vi "ziModGetNextNode.vi"(8 "Error In":errorcluster, 11 "ModHandle In":T4 {"ModHandle" format="0x%08x"; "Conn" format="0x%08x"}) -> (0 "Error Out":errorcluster, 2 "ModResults":T1, 3 "ModHandle Out":T4 {"ModHandle" format="0x%08x"; "Conn" format="0x%08x"}, 4 "NoData":bool)   [LabVIEW 2018, in "Zurich Instruments LabOne.lvlib"]
doc: "Use this device to extract the data from subscribed node, which you polled from device by ziModExecute.vi (with modal is false) or the ziModRead.vi. This allows to iterate through ModResults and return the <b>Path, the ValueType and the NoOfResults</b>. If this iterator, does not find any more data, the <b>NoData</b> flag is raised."
uses:
  Zurich Instruments LabOne.lvlib
  ziTypeModHandle.ctl
  ziTypeModResults.ctl
  Data/ziTypePollType.ctl
  ziTypeModGenericHeader.ctl
  ziLV32.dll
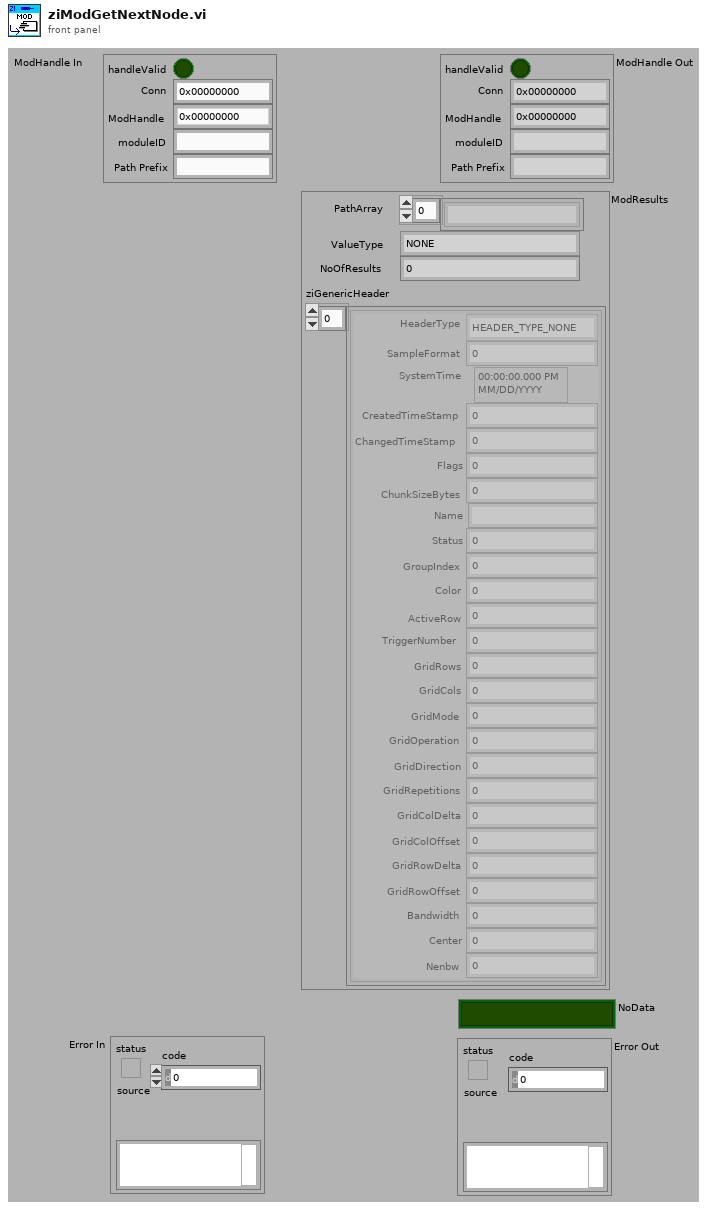
[diagram p1: front panel]
types:
  T1 = typedef "Zurich Instruments LabOne.lvlib/ziTypeModResults.ctl" = cluster{"PathArray":string[], "ValueType":T2, "NoOfResults":u64, "ziGenericHeader":T3[]}
  T2 = typedef "Zurich Instruments LabOne.lvlib/ziTypePollType.ctl" = enum16{"NONE", "DOUBLE_DATA", "INTEGER_DATA", "DEMOD_SAMPLE", "SCOPE_WAVE_HF2", "AUXIN_SAMPLE", "DIO_SAMPLE", "BYTE_ARRAY", "PWA_WAVE", "9", "10", "11", "12", "13", "14", "15", "TREE_CHANGE_DEPRI", "17", "ERROR", "19", "20", "21", "22", "23", "24", "25", "26", "27", "28", "29", "30", "31", "DOUBLE_DATA_TS", "INTEGER_DATA_TS", "34", "SCOPE_WAVE", "SCOPE_WAVE_EX", "37", "BYTE_ARRAY_TS", "39", "40", "41", "42", "43", "44", "45", "CNT_DATA", "47", "TREE_CHANGE", "49", "50", "51", "52", "53", "54", "55", "56", "57", "58", "59", "60", "61", "62", "63", "SWEEPER_DATA", "SPECTRUM_DATA", "ADVISOR_DATA", "VECTOR_DATA", "IMP_DATA"}
  T3 = typedef "Zurich Instruments LabOne.lvlib/ziTypeModGenericHeader.ctl" = cluster{"HeaderType":enum8{"HEADER_TYPE_NONE", "HEADER_TYPE_SWTRIGGER", "HEADER_TYPE_SWEEPER"}, "SampleFormat":u8, "SystemTime":timestamp, "CreatedTimeStamp":u64, "ChangedTimeStamp":u64, "Flags":u32, "ChunkSizeBytes":u64, "Name":string, "Status":u32, "GroupIndex":u32, "Color":u32, "ActiveRow":u32, "TriggerNumber":u64, "GridRows":u32, "GridCols":u32, "GridMode":u32, "GridOperation":u32, "GridDirection":u32, "GridRepetitions":u32, "GridColDelta":dbl, "GridColOffset":dbl, "GridRowDelta":dbl, "GridRowOffset":dbl, "Bandwidth":dbl, "Center":dbl, "Nenbw":dbl}
  T4 = typedef "Zurich Instruments LabOne.lvlib/ziTypeModHandle.ctl" = cluster{"handleValid":bool, "Conn":u64, "ModHandle":u64, "moduleID":string, "Path Prefix":string}
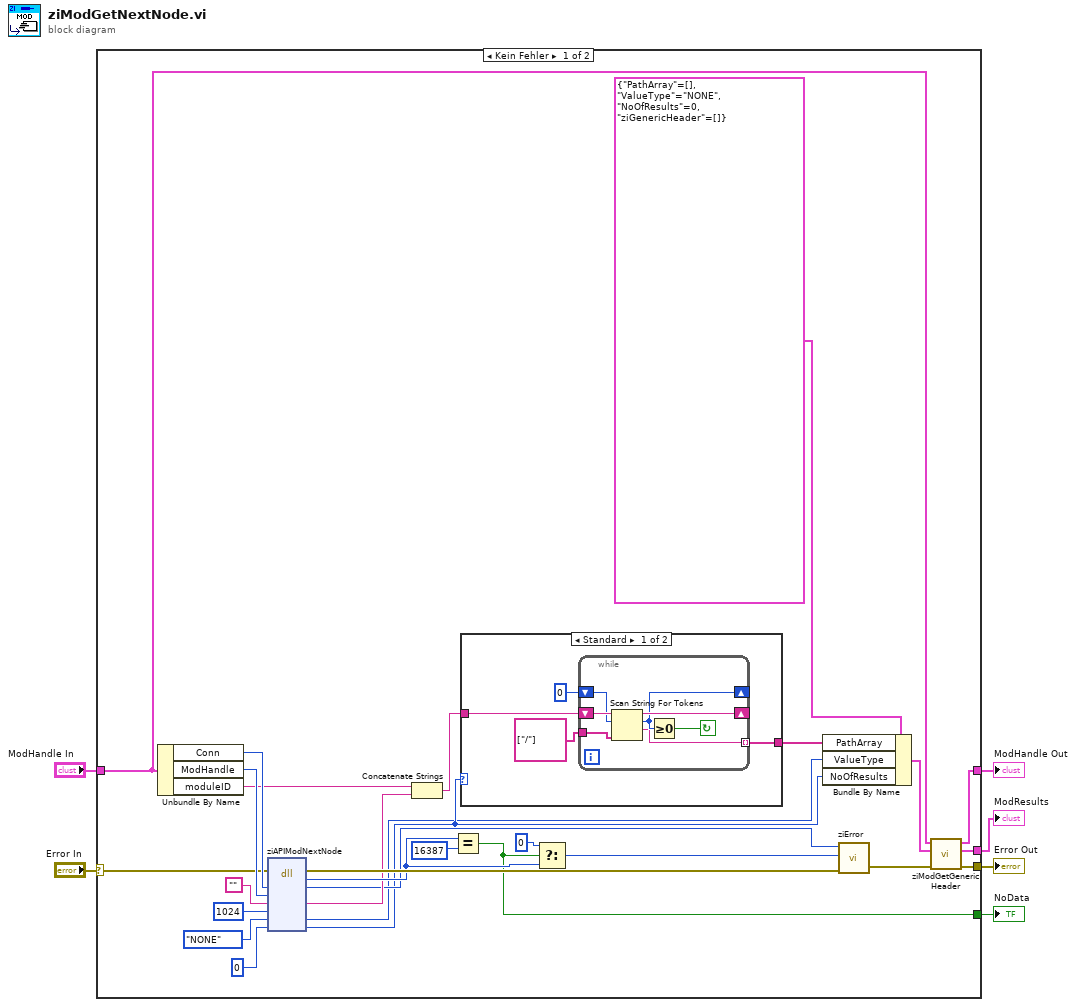
[diagram p0: block diagram]
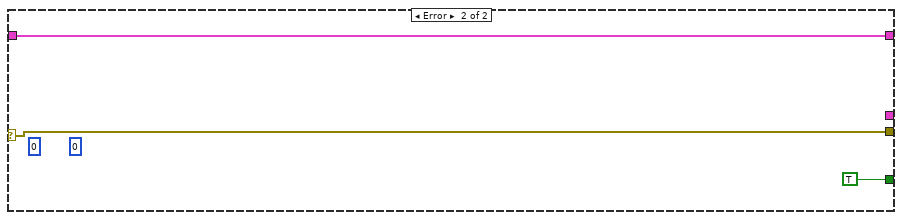
[diagram p3: hidden frame]
diagram:
  n1 = case shown="Kein Fehler" "Error In" {
    selector: "Error In" -> [w31 w45]
    tunnel: [w12 w45] -> w2
    tunnel: [w15 w47] -> w3
    tunnel: "ModHandle In" -> [w16 w47]
    tunnel: [w14 TRUE] -> w4
    tunnel: [w7 _] -> w1
    frame No Error {
      n2 = Unbundle By Name(w16) -> ("Conn"=w33:u64, "ModHandle"=w32:u64, "moduleID"=w23:string)
      n3 = dll-call lib="ziLV*.*" fn="ziAPIModNextNode"(error in=w31, "Conn"=w33, "ModHandle"=w32, "Path"="", "bufferSize"=u32 1024, "valueType"=ziTypePollType."NONE" ("ValueType"), "NoOfResults"=u64 0) -> (error out=w30:errorcluster, "return type"=w26:u32, "Conn"=w20:u64, "Path"=w22:string, "valueType"=w17:u64, "NoOfResults"=w18:u64)  [unwired: 4 in, 1 out]
      n4 = Concatenate Strings(w23, w22) -> (w21:string)
      n5 = Equal?(x=w26, y=u32 16387) -> (x = y?=w14:bool)
      n6 = case shown="Standard" w18 {
        tunnel: w21 -> [w35 _]
        tunnel: [w36 _] -> w19
        frame Default {
          n7 = while {
            shift-right: [w42] -> _
            shift-left: w35 -> [w44]
            shift-right: [w41] -> _
            shift-left: 0 ("offset past token") -> [w43]
            tunnel: [w39] -> w36 mode=indexing
            tunnel: string[] ["/"] ("delimiters (\\s,\\t,\\r,\\n)") -> [w38]
            stop <- w40 continue-if-true
            n8 = Scan String For Tokens(6:w38, 8:w43, 9:w44) -> (1:w39:string, 2:w41:i32, 3:w42:string)  [unwired: 1 in, 3 out]
            n9 = Greater Or Equal To 0?(x=w41) -> (x >= 0?=w40:bool)
          }
        }
        frame 0 {
        }
      }
      n10 = Select(t=u32 0, s=w14, f=w26) -> (s? t:f=w24:u32)
      n11 = Bundle By Name "Bundle By Name"(cluster=T1 {"PathArray"=[], "ValueType"=enum."NONE", "NoOfResults"=0, "ziGenericHeader"=[]} ("ziModResults 2"), "PathArray"=w19, "ValueType"=w17, "NoOfResults"=w18) -> (w8:T1)
      n12 = call "ziError.vi"("Conn"=w20, "ziErrorCode"=w24, "Error In"=w30) -> ("Error Out"=w13:errorcluster)  [unwired: 2 in, 1 out]
      n13 = call "ziModGetGenericHeader.vi"("Error In"=w13, "ModResults"=w8, "ModHandle In"=w16) -> ("Error Out"=w12:errorcluster, "ModResults"=w7:T1, "ModHandle Out"=w15:T4)  [unwired: 6 in]
    }
    frame Error {
      (unwired) u64 0 ("NoOfResults")
      (unwired) u64 0 ("valueType")
    }
  }
  "Error Out" <- w2
  "ModHandle Out" <- w3
  "NoData" <- w4
  "ModResults" <- w1
